vi "svx_Build Orbit and Timebase Data (N Ch - 1 Order).vi"(4 "pair index":cluster{"index 1":i32, "index 2":i32}[](array[cluster]), 5 "magnitudes info":T1[](array[typedef]) {"x-axis units" items=["Time (s)"=0, "Frequency-CB (Hz)"=1, "Frequency-CPB (Hz)"=1248, "Frequency-Arbitrary (Hz)"=2357, "Quefrency (s)"=2, "Revolutions (rev)"=3, "Order"=4, "Speed (RPM)"=11, "Speed (rad/s)"=21, "Index"=65535]; "weighting filter" items=["Linear", "A-weighting", "B-weighting", "C-weighting", "ITU-R 468-4", "Dolby", "CCITT", "C-message", "Wb", "Wc", "Wd", "We", "Wf", "Wh", "Wj", "Wk", "Wm", "AES17 20 kHz lowpass", "AES17 40 kHz lowpass", "AES17 20 kHz highpass", "AES17 40 kHz highpass"]; "dB reference [EU]" format="%.2f"; "engineering units" items=["custom..."=0, "V"=1, "A"=21, "C"=30, "pC"=31, "s"=32, "-"=29, "Pa"=2, "N"=20, "g"=3, "m/s^2"=4, "m/s"=5, "m"=6, "mm/s"=12, "mm"=13, "micron/s"=14, "micron"=15, "in/s^2"=7, "in/s"=8, "in"=9, "mil/s"=10, "mil"=11, "rad/s^2"=16, "rad/s"=17, "rad"=18, "deg/s^2"=26, "deg/s"=27, "deg"=28, "RPM"=22, "cycle/s^2"=23, "Hz"=24, "cycle"=25, "strain"=19]; "spectral info"."window" items=["None "=0, "Hanning"=1, "Hamming"=2, "Blackman-Harris"=3, "Exact Blackman"=4, "Blackman"=5, "Flat Top"=6, "4 Term B-Harris "=7, "7 Term B-Harris"=8, "Low Sidelobe"=9, "Force - Exponential"=10, "Gaussian"=62]}, 6 "channel properties":T7[](array[typedef]) {"probe angle [deg]" max=360; "direction" items=["CCW", "CW"]}, 7 "order":dbl, 8 "error in (no error)":errorcluster, 9 "actual samples/rev":dbl=1.0 format="%.2f", 10 "interpolated pulse positions[s]":dbl[](array[numeric]) format="%.2f", 11 "order data":dbl[][](array[numeric])) -> (0 "error out":errorcluster, 3 "orbit/timebase plot":T8(array[cluster]))   [LabVIEW 2017]
uses:
  <vilib>/addons/Sound and Vibration/Order Analysis/Data Presentation/SubVIs/OAT MCM Channel Property.ctl
  <vilib>/addons/_NISVFA/_Shared subVIs/Controls/svc_Spectrum Info.ctl
  <vilib>/addons/_NISVFA/_Shared subVIs/Controls/svc_X-Axis Units.ctl
  <vilib>/addons/_NISVFA/_Shared subVIs/Controls/svc_Spectrum Type.ctl
  <vilib>/addons/_NISVFA/_Shared subVIs/Controls/svc_Engineering Units Text Ring.ctl
  <vilib>/addons/_NISVFA/_Shared subVIs/Controls/svc_Weighting Filter Text Ring.ctl
  <vilib>/addons/_NISVFA/_Shared subVIs/Controls/svc_Complimentary Spectrum Units.ctl
  <vilib>/addons/Sound and Vibration/Order Analysis/Misc/SVMS Attribute.ctl
  <vilib>/addons/_NISVFA/_Shared subVIs/Controls/NI Channel Properties.ctl
  <vilib>/addons/_NISVFA/_Shared subVIs/Common/svc_Get Weighting Enum and Labels.vi
  <vilib>/addons/_NISVFA/_Shared subVIs/Common/svc_Unit Label Lexical Class.vi
  <vilib>/addons/_NISVFA/_Shared subVIs/Common/svc_Engineering Units to Unit Label.vi
  <vilib>/addons/_NISVFA/_Shared subVIs/Common/svc_Format Value (DBL).vi
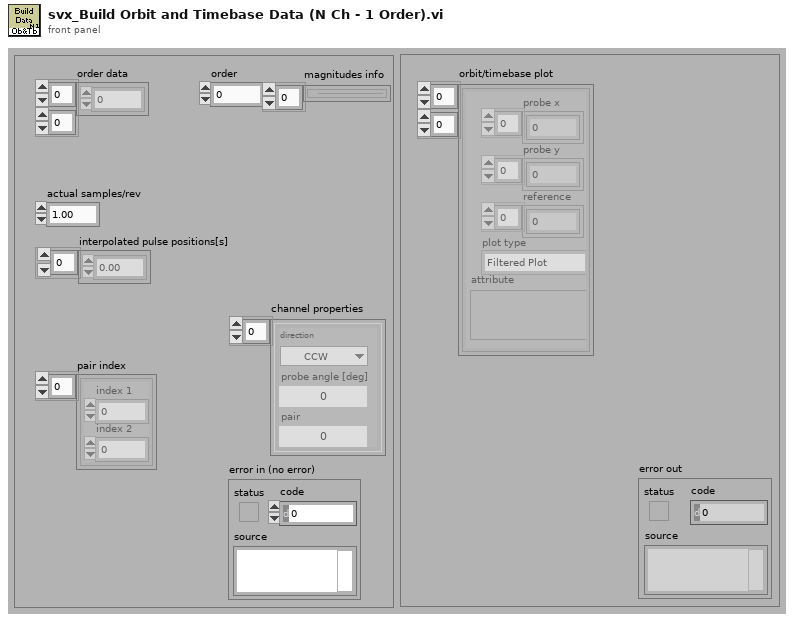
[diagram p1: front panel]
types:
  T1 = typedef "svc_Spectrum Info.ctl" = cluster{"channel name":string, "description":string, "x-axis units":T2, "spectral info":cluster{"spectrum type":T3, "linear/dB":enum16{"linear", "dB"}, "window":u16, "window size":i32, "FFT size":i32}, "engineering units":T4, "custom label":string, "dB reference [EU]":dbl, "peak units":enum16{"rms", "peak", "peak-peak"}, "weighting filter":T5, "spectral density?":bool, "unit label":string, "spectrum skewed?":bool, "complimentary spectrum units":T6}
  T2 = typedef "svc_X-Axis Units.ctl" = u16
  T3 = typedef "svc_Spectrum Type.ctl" = enum16{"FFT Spectrum [complex]", "Amplitude [Magnitude]", "Power [Magnitude^2]", "Cross Spectrum [complex]", "Frequency Response [Complex]"}
  T4 = typedef "svc_Engineering Units Text Ring.ctl" = u16
  T5 = typedef "svc_Weighting Filter Text Ring.ctl" = u16
  T6 = typedef "svc_Complimentary Spectrum Units.ctl" = enum16{"none", "radians", "degrees", "cycles", "imaginary"}
  T7 = typedef "OAT MCM Channel Property.ctl" = cluster{"direction":u16, "probe angle [deg]":u16, "pair":u16}
  T8 = cluster{"probe x":dbl[], "probe y":dbl[], "reference":dbl[], "plot type":enum16{"Filtered Plot", "Unfiltered Plot"}, "attribute":variant}[][]
  T9 = cluster{"X":dbl[], "Y":dbl[], "reference":dbl[], "plot type":enum16{"Filtered Plot", "Unfiltered Plot"}, "attribute":variant}
  T10 = typedef "NI Channel Properties.ctl" = u16
  T11 = typedef "SVMS Attribute.ctl" = u16
  T12 = cluster{"X":dbl[], "Y":dbl[], "reference":dbl[], "plot type":enum16{"Filtered Plot", "Unfiltered Plot"}, "attribute":variant}[]
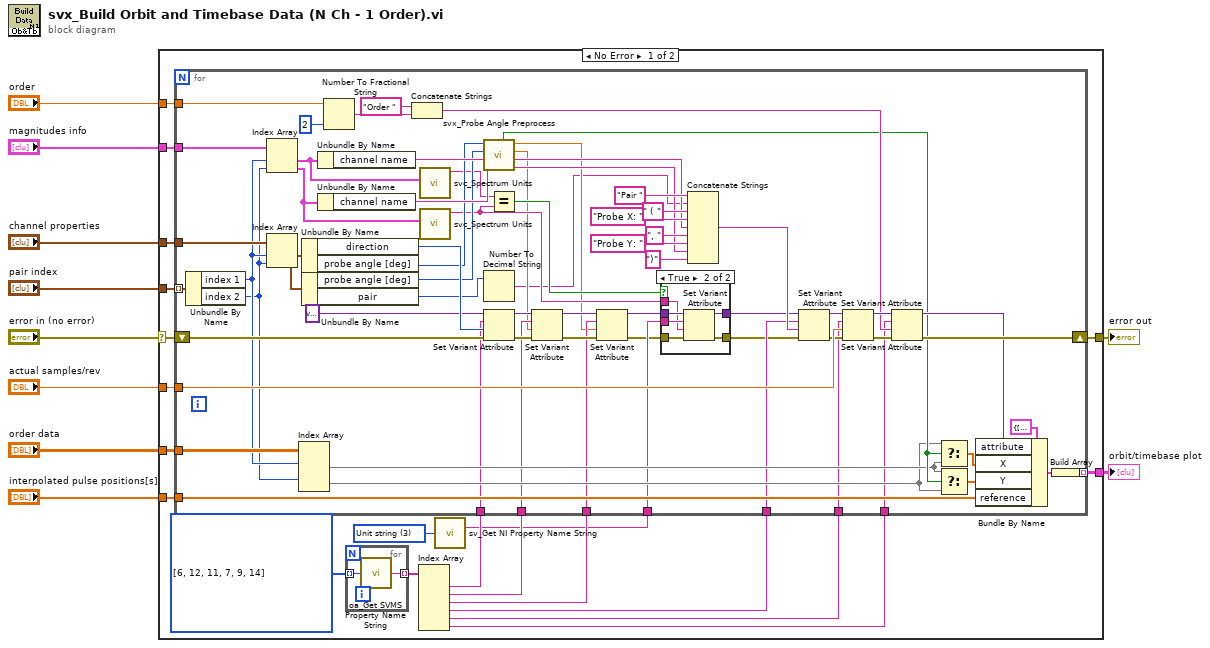
[diagram p0: block diagram]
diagram:
  n1 = case shown="No Error" "error in (no error)" {
    selector: "error in (no error)" -> [w28 w110]
    tunnel: "channel properties" -> [w30 _]
    tunnel: "order data" -> [w29 _]
    tunnel: [w27 w110] -> w8
    tunnel: "actual samples/rev" -> [w26 _]
    tunnel: "order" -> [w25 _]
    tunnel: "interpolated pulse positions[s]" -> [w24 _]
    tunnel: "magnitudes info" -> [w23 _]
    tunnel: [w22 _] -> w2
    tunnel: "pair index" -> [w21 _]
    frame No Error {
      w12 = T10 3 items=["Channel name", "Channel description", "Axis label", "Unit string", "Waveform X-axis label", "Waveform X-axis unit string", "x0", "dx", "Number of samples", "X channel", "Filter settled", "dB reference", "Window", "Window parameter", "Window size", "FFT size", "Peak units", "Spectrum type", "Magnitude scale", "Spectral density", "Sensor sensitivity (mV/EU)", "X-axis dimension", "LabVIEW datatype", "Function type", "Function subtype", "X values", "Independent channel", "Column index", "Collection name", "Collection ID", "X Columns", "Phase unwrapped", "Sensor type", "Sensor maximum", "Averaging mode"] ("property")
      w20 = T11[] [6, 12, 11, 7, 9, 14] items=["Pulse / Revolution", "Slope", "Threshold", "Hysteresis", "Order", "Reference Label", "Rotation Direction", "Pair String", "Polar Plot Type", "Sample Per Revolution", "Probe Angle", "Probe Angle X", "Probe Angle Y", "X Axis Unit", "OTB Plot Type"]
      n2 = for {
        tunnel: w20 -> [w32] mode=indexing
        tunnel: [w31] -> w19 mode=indexing
        n3 = call <vilib>:"oa_Get SVMS Property Name String.vi"("attribute"=w32) -> ("attribute name"=w31:string)  [unwired: 4 in]
      }
      n4 = Index Array(array=w19) -> (element #1=w18:string, element #2=w17:string, element #3=w16:string, element #4=w15:string, element #5=w14:string, element #6=w13:string)  [unwired: 6 in]
      n5 = call <vilib>:"sv_Get NI Property Name String.vi"("property"=w12) -> ("TDMS property name"=w11:string)  [unwired: 13 in, 1 out]
      n6 = for {
        shift-right: [w101] -> w27
        shift-left: w28 -> [w69]
        tunnel: w26 -> [w100]
        tunnel: w25 -> [w99]
        tunnel: w24 -> [w98]
        tunnel: [w72] -> w22 mode=indexing
        tunnel: w21 -> [w71] mode=indexing
        tunnel: w30 -> [w70]
        tunnel: w23 -> [w66]
        tunnel: w29 -> [w65]
        tunnel: w18 -> [w51]
        tunnel: w17 -> [w50]
        tunnel: w16 -> [w49]
        tunnel: w15 -> [w48]
        tunnel: w14 -> [w47]
        tunnel: w13 -> [w46]
        tunnel: w11 -> [w40]
        n7 = Unbundle By Name(w71) -> ("index 1"=w64:i32, "index 2"=w63:i32)
        n8 = Index Array(array=w66, index #1=w64, index #2=w63) -> (element #1=w45:T1, element #2=w44:T1)
        n9 = Index Array(array=w70, index #1=w64, index #2=w63) -> (element #1=w68:T7, element #2=w67:T7)
        n10 = Index Array(array=w65, index (row) #1=w64, index (row) #2=w63) -> (element #1=w54:dbl[], element #2=w52:dbl[])  [unwired: 2 in]
        n11 = Unbundle By Name(w68) -> ("direction"=w93:u16, "probe angle [deg]"=w60:u16)
        n12 = Unbundle By Name(w67) -> ("probe angle [deg]"=w59:u16, "pair"=w74:u16)
        n13 = Unbundle By Name(w45) -> ("channel name"=w62:string)
        n14 = Unbundle By Name(w44) -> ("channel name"=w61:string)
        n15 = Number To Fractional String(number=w99, precision (6)=i16 2) -> (F-format string=w83:string)  [unwired: 2 in]
        n16 = Concatenate Strings("Order " ("string"), w83) -> (w81:string)
        n17 = call <vilib>:"svc_Spectrum Units.vi"("spectrum info in"=w45) -> ("unit label"=w43:string)  [unwired: 3 in, 3 out]
        n18 = call <vilib>:"svc_Spectrum Units.vi"("spectrum info in"=w44) -> ("unit label"=w41:string)  [unwired: 3 in, 3 out]
        n19 = call <vilib>:"svx_Probe Angle Preprocess.vi"("channel name Y"=w61, "channel name X"=w62, "Y"=w59, "X"=w60) -> ("actual Y"=w57:string, "actual X"=w58:string, "Y"=w34:dbl, "X"=w35:dbl, "switched?"=w55:bool)  [unwired: 3 in]
        n20 = Number To Decimal String(number=w74) -> (decimal integer string=w33:string)  [unwired: 1 in]
        n21 = Set Variant Attribute(Variant=variant ("variant"), name=w51, value=w93, error in=w69) -> (Variant out=w97:variant, error out=w96:errorcluster)  [unwired: 1 out]
        n22 = Equal?(x=w43, y=w41) -> (x = y?=w42:bool)
        n23 = Set Variant Attribute(Variant=w97, name=w50, value=w34, error in=w96) -> (Variant out=w94:variant, error out=w95:errorcluster)  [unwired: 1 out]
        n24 = Set Variant Attribute(Variant=w94, name=w49, value=w35, error in=w95) -> (Variant out=w39:variant, error out=w38:errorcluster)  [unwired: 1 out]
        n25 = case shown="True" w42 {
          tunnel: w38 -> [w102 w109]
          tunnel: w39 -> [w103 w108]
          tunnel: [w102 w107] -> w36
          tunnel: [w103 w106] -> w37
          tunnel: w40 -> [_ w105]
          tunnel: w41 -> [_ w104]
          frame False {
          }
          frame True {
            n26 = Set Variant Attribute(Variant=w108, name=w105, value=w104, error in=w109) -> (Variant out=w106:variant, error out=w107:errorcluster)  [unwired: 1 out]
          }
        }
        n27 = Concatenate Strings("Pair " ("string"), w33, " ( " ("string"), "Probe X: " ("string"), w58, ", " ("string"), "Probe Y: " ("string"), w57, ")" ("string")) -> (w73:string)
        n28 = Set Variant Attribute(Variant=w37, name=w48, value=w73, error in=w36) -> (Variant out=w91:variant, error out=w90:errorcluster)  [unwired: 1 out]
        n29 = Set Variant Attribute(Variant=w91, name=w47, value=w100, error in=w90) -> (Variant out=w88:variant, error out=w89:errorcluster)  [unwired: 1 out]
        n30 = Set Variant Attribute(Variant=w88, name=w46, value=w81, error in=w89) -> (Variant out=w86:variant, error out=w101:errorcluster)  [unwired: 1 out]
        n31 = Select(t=w52, s=w55, f=w54) -> (s? t:f=w56:dbl[])
        n32 = Select(t=w54, s=w55, f=w52) -> (s? t:f=w53:dbl[])
        n33 = Bundle By Name(cluster=T9 {"X"=[], "Y"=[], "reference"=[], "plot type"=enum."Filtered Plot", "attribute"=variant} ("orbit plot 2"), "attribute"=w86, "X"=w56, "Y"=w53, "reference"=w98) -> (w85:T9)
        n34 = Build Array(w85) -> (w72:T12)
      }
    }
    frame Error {
    }
  }
  "orbit/timebase plot" <- w2
  "error out" <- w8
